vi "TableCnt.vi"(7 "cnt":T1, 8 "error in":errorcluster caption="에러 입력(에러 없음)", 10 "appended array":string[](array[string]), 11 "table_result":refnum<vi>) -> (0 "error out":errorcluster, 3 "Item Names":string[][](array[string]))   [LabVIEW 2019]
uses:
  cmd_tablecnt.ctl
  <vilib>/Utility/miscctls.llb/LVRowAndColumnTypeDef.ctl
  _ctrl/rw.ctl
  Durability/common/Global 1.vi
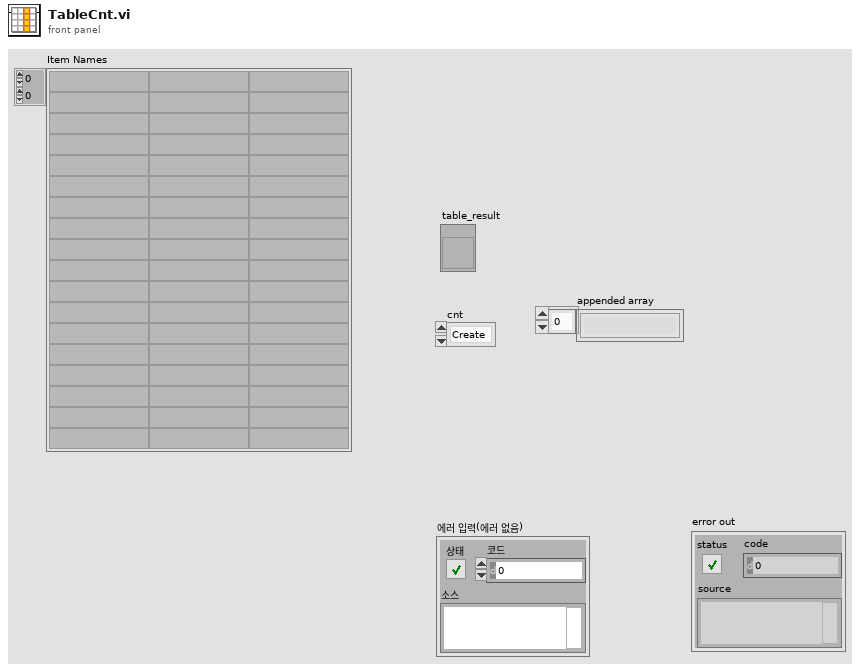
[diagram p1: front panel]
types:
  T1 = typedef "cmd_tablecnt.ctl" = enum16{"Create", "Inital", "Write", "Default"}
  T2 = typedef "LVRowAndColumnTypeDef.ctl" = cluster{"Row":i32, "Column":i32}
  T3 = typedef "rw.ctl" = enum16{"read", "write"}
  T4 = typedef "Test Mode.ctl" = enum32{"저항부하", "캐패시터부하", "B수명 - 1", "B수명 - 2", "B수명 - 3", "저전압모드 동작검사", "저전압모드 접촉저항", "고전압모드 동작검사"}
  T5 = typedef "Testing-info.ctl" = cluster{"전체채널수":u8, "현재채널번호":u8, "Irms":dbl, "입력전압":dbl, "입력전류":dbl, "출력전압":dbl, "출력전류":dbl, "온도":dbl, "제어단 단선":bool, "제어단 단락":bool, "제어단 특성변화":bool, "출력단 단선":bool, "출력단 단락":bool, "출력단 특성변화":bool, "출력단 전압":bool, "카운트 일치":bool, "Irms 판정":bool, "온도":bool, "테스트 회수":u32, "TestType":T6, "현재회수":u32, "Ch selection":cluster{"1ch":bool, "2ch":bool, "3ch":bool, "4ch":bool, "5ch":bool, "6ch":bool}, "반복":u32, "Path":path, "파일생성주기":u32, "start time":dbl, "stop time":dbl, "현재반복회수":u32, "NG":cluster{"입출력 카운트":bool, "출력전류RMS":bool}}
  T6 = typedef "sequence_single.ctl" = enum16{"Register", "RC", "B1", "B2", "B3", "Oper_LV", "Oper_HV", "ContR_LV"}
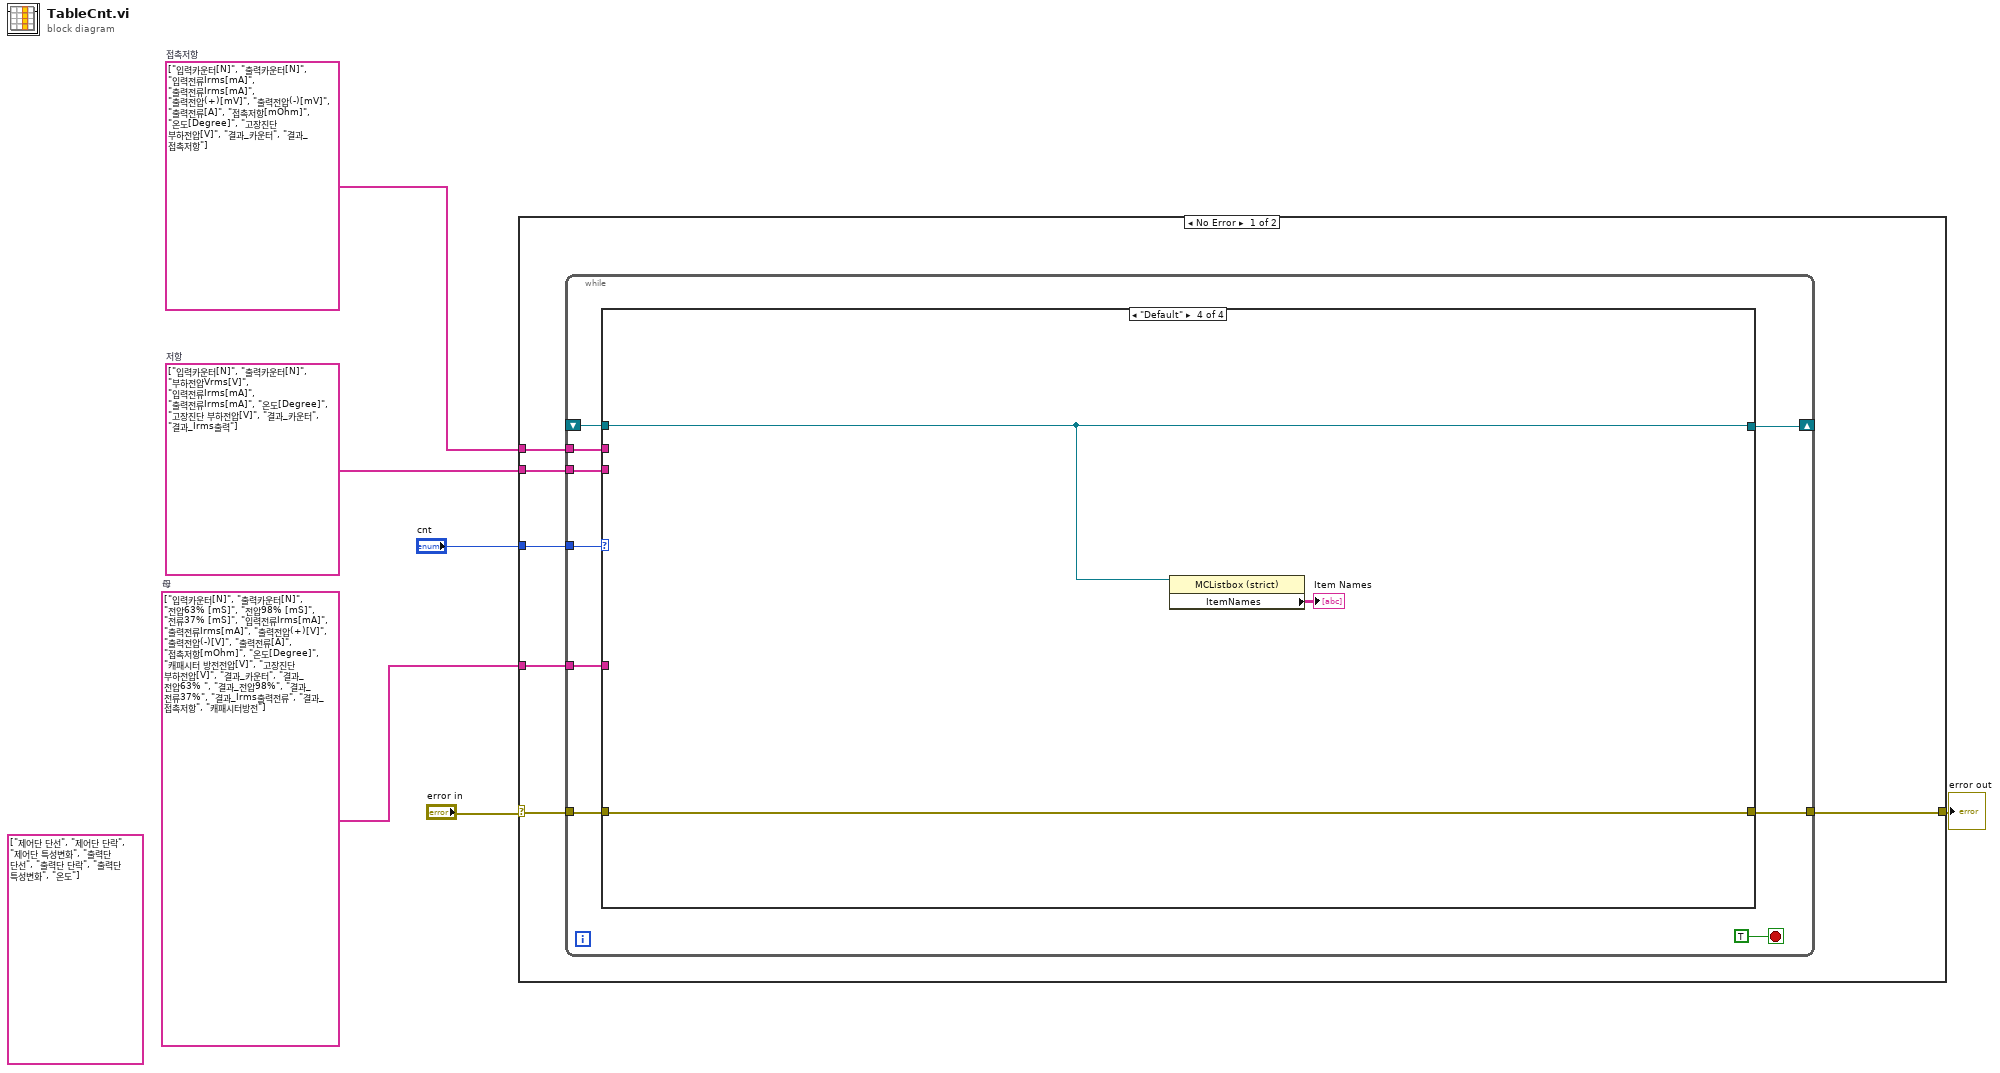
[diagram p0: block diagram]
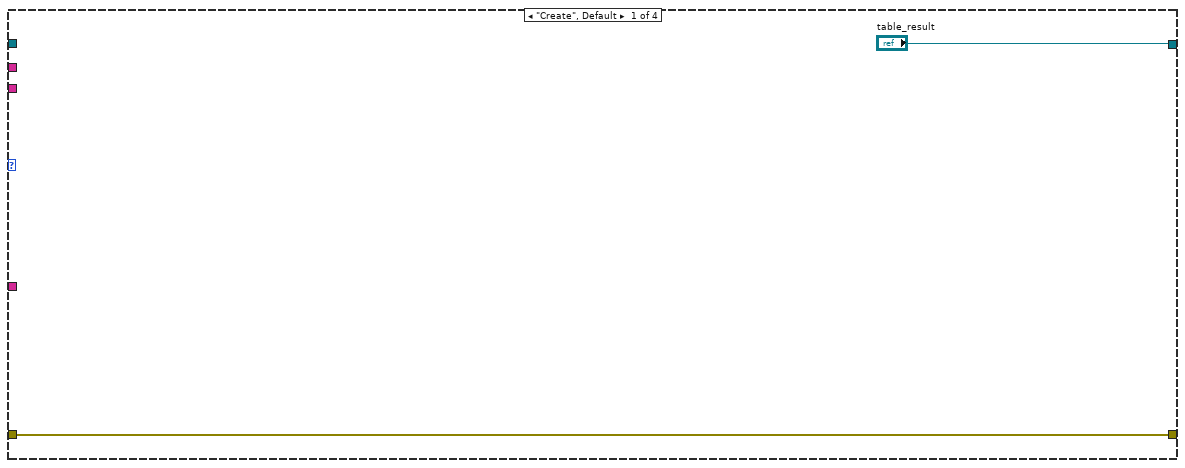
[diagram p2: hidden frame]
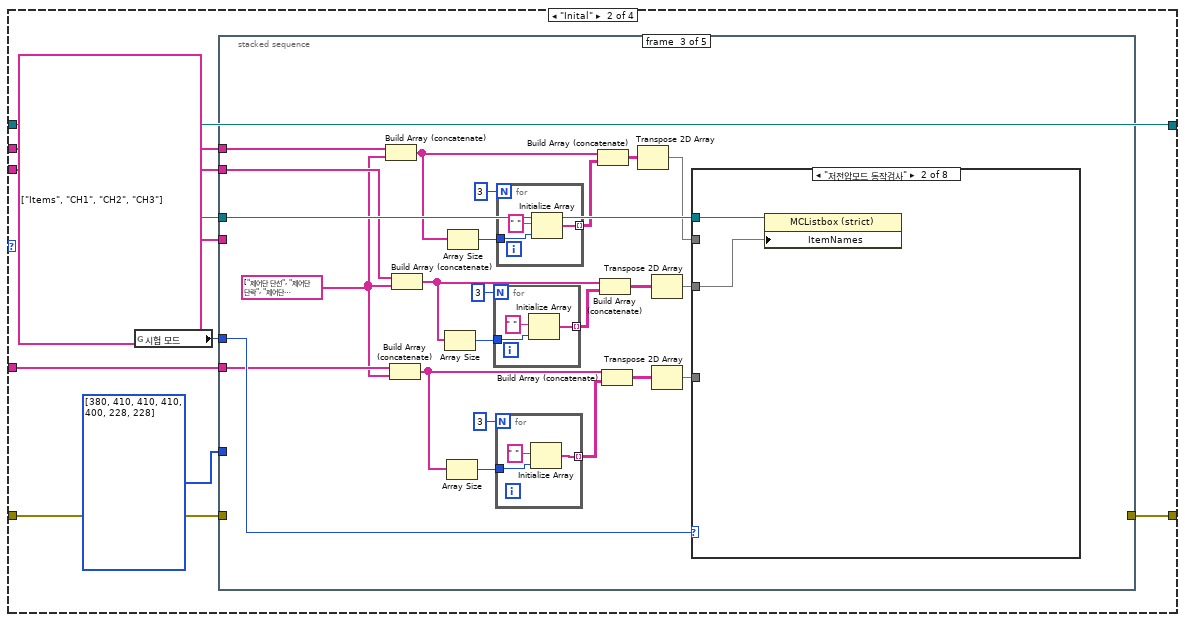
[diagram p3: hidden frame]
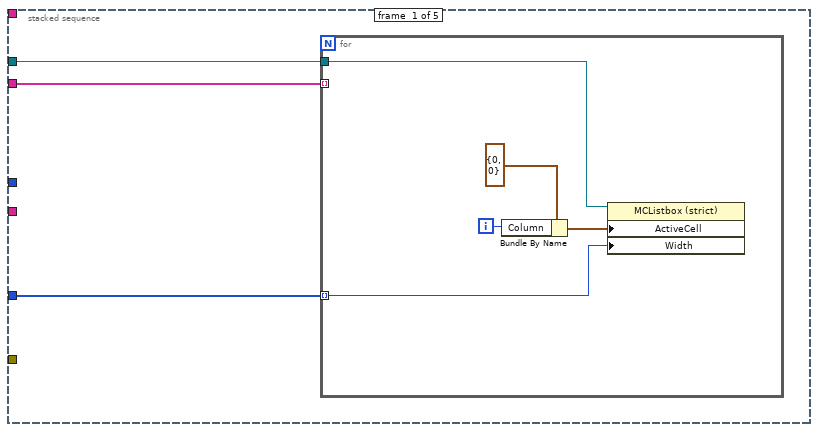
[diagram p4: hidden frame]
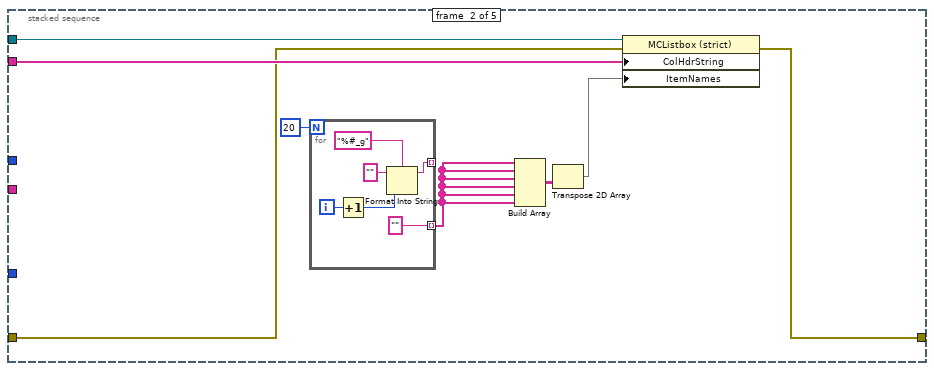
[diagram p5: hidden frame]
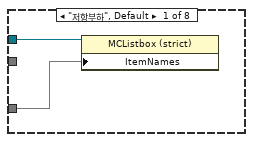
[diagram p6: hidden frame]
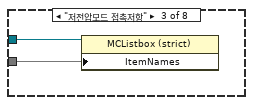
[diagram p7: hidden frame]
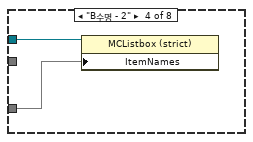
[diagram p8: hidden frame]
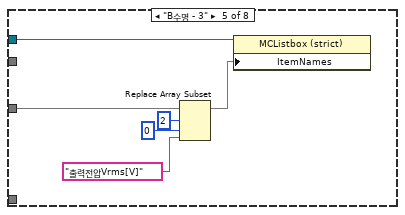
[diagram p9: hidden frame]
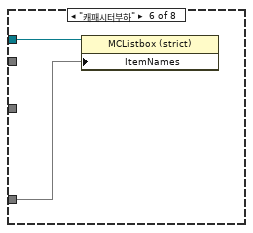
[diagram p10: hidden frame]
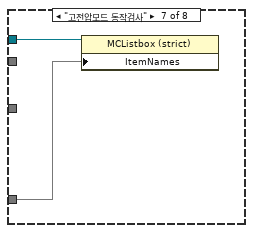
[diagram p11: hidden frame]
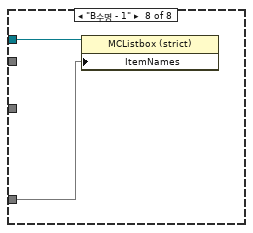
[diagram p12: hidden frame]
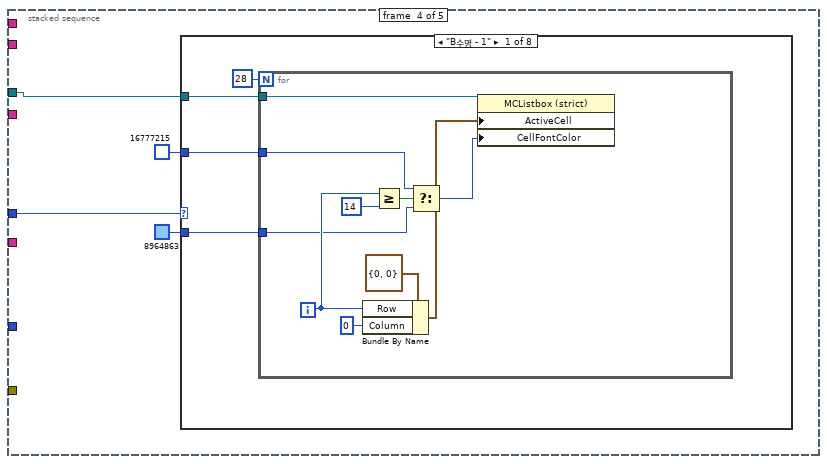
[diagram p13: hidden frame]
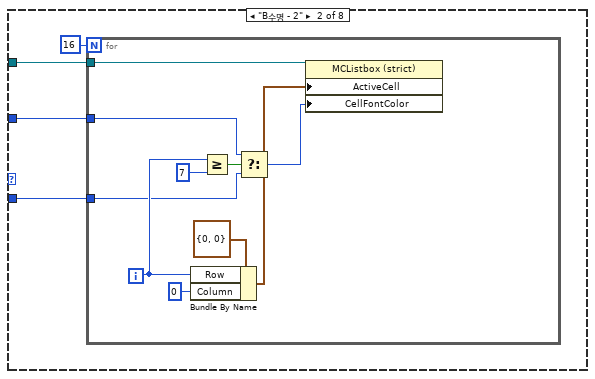
[diagram p14: hidden frame]
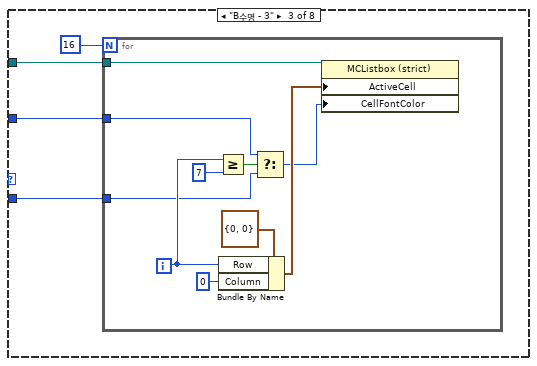
[diagram p15: hidden frame]
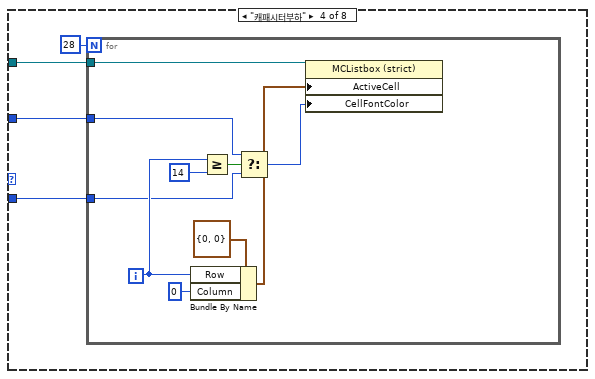
[diagram p16: hidden frame]
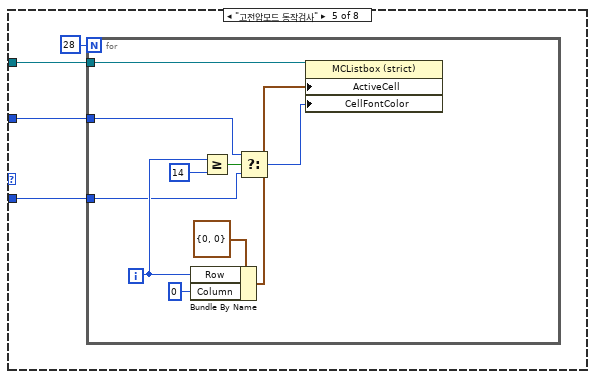
[diagram p17: hidden frame]
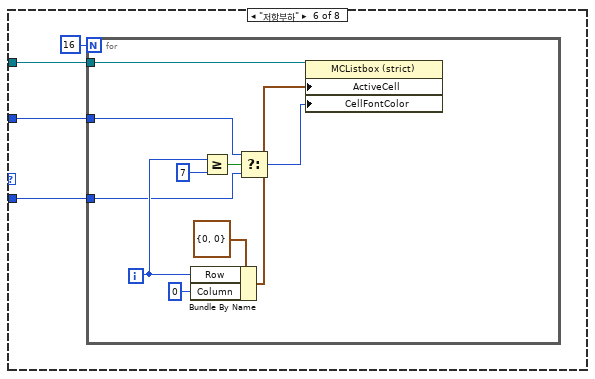
[diagram p18: hidden frame]
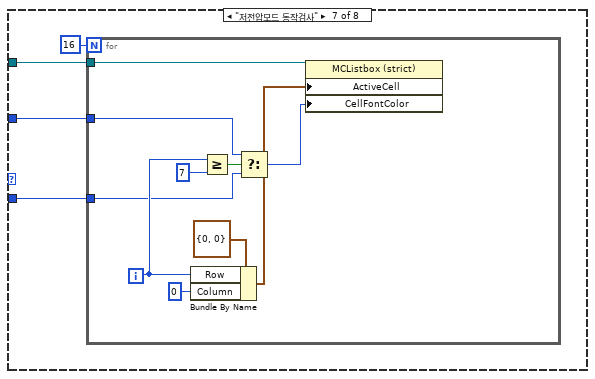
[diagram p19: hidden frame]
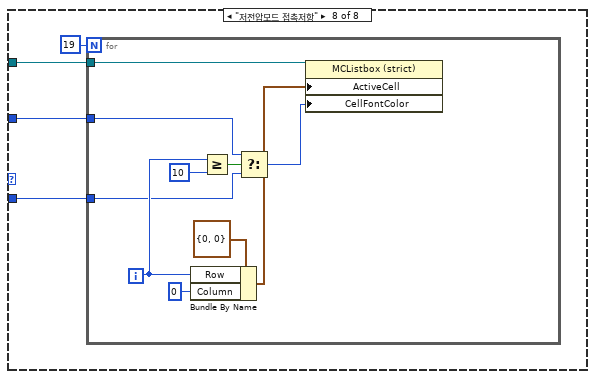
[diagram p20: hidden frame]
diagram:
  (unwired) string[] ["제어단 단선", "제어단 단락", "제어단 특성변화", "출력단 단선", "출력단 단락", "출력단 특성변화", "온도"] ("Column Header Strings[]")
  w1 = string[] ["입력카운터[N]", "출력카운터[N]", "입력전류Irms[mA]", "출력전류Irms[mA]", "출력전압(+)[mV]", "출력전압(-)[mV]", "출력전류[A]", "접촉저항[mOhm]", "온도[Degree]", "고장진단 부하전압[V]", "결과_카운터", "결과_접촉저항"]  # 접촉저항
  w2 = string[] ["입력카운터[N]", "출력카운터[N]", "전압63% [mS]", "전압98% [mS]", "전류37% [mS]", "입력전류Irms[mA]", "출력전류Irms[mA]", "출력전압(+)[V]", "출력전압(-)[V]", "출력전류[A]", "접촉저항[mOhm]", "온도[Degree]", "캐패시터 방전전압[V]", "고장진단 부하전압[V]", "결과_카운터", "결과_전압63% ", "결과_전압98%", "결과_전류37%", "결과_Irms출력전류", "결과_접촉저항", "캐패시터방전"]  # 母
  w3 = string[] ["입력카운터[N]", "출력카운터[N]", "부하전압Vrms[V]", "입력전류Irms[mA]", "출력전류Irms[mA]", "온도[Degree]", "고장진단 부하전압[V]", "결과_카운터", "결과_Irms출력"]  # 저항
  n1 = case shown="No Error" "error in" {
    selector: "error in" -> [w12 w443]
    tunnel: "cnt" -> [w11 _]
    tunnel: [w10 w443] -> w5
    tunnel: w3 -> [w9 _]
    tunnel: w2 -> [w8 _]
    tunnel: w1 -> [w7 _]
    frame No Error {
      n2 = while {
        tunnel: w12 -> [w17]
        tunnel: w11 -> [w20]
        shift-right: [w19] -> _
        shift-left: _ -> [w18]
        tunnel: [w16] -> w10
        tunnel: w9 -> [w15]
        tunnel: w8 -> [w14]
        tunnel: w7 -> [w13]
        stop <- TRUE stop-if-true
        n3 = case shown="\"Default\"" w20 {
          tunnel: ["table_result" w28 w227 w441] -> w19
          tunnel: w18 -> [_ w28 w227 w441]
          tunnel: w17 -> [w23 w31 _ w442]
          tunnel: [w23 w30 _ w442] -> w16
          tunnel: w15 -> [_ w26 _ _]
          tunnel: w14 -> [_ w25 _ _]
          tunnel: w13 -> [_ w24 _ _]
          frame "Create", Default {
          }
          frame "Inital" {
            n4 = global read "Global 1.vi" "시험 모드"() -> (w27:T4)
            n5 = stacked-sequence {
              tunnel: w28 -> [w34 w48 w78 w111 w225]
              tunnel: string[] ["Items", "CH1", "CH2", "CH3"] ("Column Header Strings[]") -> [w35 w47 _ _ _]
              tunnel: w31 -> [_ w46 _ _ _]
              tunnel: [_ w45 _ _ _] -> w30
              tunnel: u32[] [380, 410, 410, 410, 400, 228, 228] -> [w33 _ _ _ _]
              tunnel: w27 -> [_ _ w73 w110 _]
              tunnel: w26 -> [_ _ w64 _ _]
              tunnel: w25 -> [_ _ w63 _ _]
              tunnel: w24 -> [_ _ w61 _ _]
              frame #0 {
                n6 = for {
                  tunnel: w35 -> [_] mode=indexing
                  tunnel: w34 -> [w40]
                  tunnel: w33 -> [w37] mode=indexing
                  i -> [w36]
                  n7 = Bundle By Name(cluster=T2 {"Row"=0, "Column"=0} ("Active Cell:Active Cell"), "Column"=w36) -> (w38:T2)
                  n8 = property class="MCListbox (strict)"(reference=w40, "ActiveCell"=w38, "Width"=w37) -> ()  [unwired: 1 in, 2 out]
                }
              }
              frame #1 {
                n9 = for {
                  N: 20 -> [_]
                  tunnel: [w51] -> _ mode=indexing
                  tunnel: [""] -> w41 mode=indexing
                  i -> [w54]
                  n10 = Increment(x=w54) -> (x+1=w50:i32)
                  n11 = Format Into String(format string="%#_g" ("포맷 문자열"), initial string="" ("초기 문자열"), w50) -> (resulting string=w51:string)  [unwired: 1 in, 1 out]
                }
                n12 = Build Array(w41, w41, w41, w41, w41, w41) -> (w43:string[][])
                n13 = Transpose 2D Array(2D array=w43) -> (transposed array=w42:string[][])
                n14 = property class="MCListbox (strict)"(reference=w48, error in=w46, "ColHdrString"=w47, "ItemNames"=w42) -> (error out=w45:errorcluster)  [unwired: 1 out]
              }
              frame #2 {
                w62 = string[] ["제어단 단선", "제어단 단락", "제어단 특성변화", "출력단 단선", "출력단 단락", "출력단 특성변화", "온도"] ("Column Header Strings[]")
                n15 = Build Array (concatenate)(w61, w62) -> (w58:string[])
                n16 = Build Array (concatenate)(w63, w62) -> (w70:string[])
                n17 = Build Array (concatenate)(w64, w62) -> (w66:string[])
                n18 = Array Size(array=w66) -> (size(s)=w68:i32)
                n19 = Array Size(array=w70) -> (size(s)=w72:i32)
                n20 = Array Size(array=w58) -> (size(s)=w60:i32)
                n21 = for {
                  N: 3 -> [_]
                  tunnel: w68 -> [w83]
                  tunnel: [w82] -> w65 mode=indexing
                  n22 = Initialize Array(" ", w83) -> (w82:string[])
                }
                n23 = for {
                  N: 3 -> [_]
                  tunnel: w72 -> [w86]
                  tunnel: [w85] -> w69 mode=indexing
                  n24 = Initialize Array(" ", w86) -> (w85:string[])
                }
                n25 = for {
                  N: 3 -> [_]
                  tunnel: w60 -> [w80]
                  tunnel: [w79] -> w57 mode=indexing
                  n26 = Initialize Array(" ", w80) -> (w79:string[])
                }
                n27 = Build Array (concatenate)(w58, w57) -> (w56:string[][])
                n28 = Build Array (concatenate)(w66, w65) -> (w75:string[][])
                n29 = Build Array (concatenate)(w70, w69) -> (w74:string[][])
                n30 = Transpose 2D Array(2D array=w56) -> (transposed array=w55:string[][])
                n31 = Transpose 2D Array(2D array=w75) -> (transposed array=w77:string[][])
                n32 = Transpose 2D Array(2D array=w74) -> (transposed array=w76:string[][])
                n33 = case shown="\"저전압모드 동작검사\"" w73 {
                  tunnel: w78 -> [w89 w91 w93 w95 w101 w103 w105 w107]
                  tunnel: w77 -> [w88 w90 _ w94 w100 _ _ _]
                  tunnel: w76 -> [_ _ _ _ _ w102 w104 w106]
                  tunnel: w55 -> [_ _ w92 _ _ _ _ _]
                  frame "저항부하", Default {
                    n34 = property class="MCListbox (strict)"(reference=w89, "ItemNames"=w88) -> ()  [unwired: 1 in, 2 out]
                  }
                  frame "저전압모드 동작검사" {
                    n35 = property class="MCListbox (strict)"(reference=w91, "ItemNames"=w90) -> ()  [unwired: 1 in, 2 out]
                  }
                  frame "저전압모드 접촉저항" {
                    n36 = property class="MCListbox (strict)"(reference=w93, "ItemNames"=w92) -> ()  [unwired: 1 in, 2 out]
                  }
                  frame "B수명 - 2" {
                    n37 = property class="MCListbox (strict)"(reference=w95, "ItemNames"=w94) -> ()  [unwired: 1 in, 2 out]
                  }
                  frame "B수명 - 3" {
                    n38 = Replace Array Subset(array=w100, new element="출력전압Vrms[V]", index (row)=2, index (col)=0 ("disabled index (col)")) -> (w99:string[][])
                    n39 = property class="MCListbox (strict)"(reference=w101, "ItemNames"=w99) -> ()  [unwired: 1 in, 2 out]
                  }
                  frame "캐패시터부하" {
                    n40 = property class="MCListbox (strict)"(reference=w103, "ItemNames"=w102) -> ()  [unwired: 1 in, 2 out]
                  }
                  frame "고전압모드 동작검사" {
                    n41 = property class="MCListbox (strict)"(reference=w105, "ItemNames"=w104) -> ()  [unwired: 1 in, 2 out]
                  }
                  frame "B수명 - 1" {
                    n42 = property class="MCListbox (strict)"(reference=w107, "ItemNames"=w106) -> ()  [unwired: 1 in, 2 out]
                  }
                }
              }
              frame #3 {
                n43 = case shown="\"B수명 - 1\"" w110 {
                  tunnel: w111 -> [w115 w129 w143 w157 w171 w185 w199 w213]
                  tunnel: u32 16777215 -> [w113 w127 w141 w155 w169 w183 w197 w211]
                  tunnel: u32 8964863 -> [w112 w126 w140 w154 w168 w182 w196 w210]
                  frame "B수명 - 1" {
                    n44 = for {
                      N: 28 -> [_]
                      tunnel: w115 -> [w125]
                      tunnel: w113 -> [w117]
                      tunnel: w112 -> [w116]
                      i -> [w121]
                      n45 = Bundle By Name(cluster=T2 {"Row"=0, "Column"=0} ("Active Cell:Active Cell"), "Row"=w121, "Column"=0) -> (w123:T2)
                      n46 = Greater Or Equal?(x=w121, y=14 ("x")) -> (x >= y?=w119:bool)
                      n47 = Select(t=w117, s=w119, f=w116) -> (s? t:f=w118:u32)
                      n48 = property class="MCListbox (strict)"(reference=w125, "ActiveCell"=w123, "CellFontColor"=w118) -> ()  [unwired: 1 in, 2 out]
                    }
                  }
                  frame "B수명 - 2" {
                    n49 = for {
                      N: 16 -> [_]
                      tunnel: w129 -> [w139]
                      tunnel: w127 -> [w131]
                      tunnel: w126 -> [w130]
                      i -> [w135]
                      n50 = Bundle By Name(cluster=T2 {"Row"=0, "Column"=0} ("Active Cell:Active Cell"), "Row"=w135, "Column"=0) -> (w137:T2)
                      n51 = Greater Or Equal?(x=w135, y=7 ("x")) -> (x >= y?=w133:bool)
                      n52 = Select(t=w131, s=w133, f=w130) -> (s? t:f=w132:u32)
                      n53 = property class="MCListbox (strict)"(reference=w139, "ActiveCell"=w137, "CellFontColor"=w132) -> ()  [unwired: 1 in, 2 out]
                    }
                  }
                  frame "B수명 - 3" {
                    n54 = for {
                      N: 16 -> [_]
                      tunnel: w143 -> [w153]
                      tunnel: w141 -> [w145]
                      tunnel: w140 -> [w144]
                      i -> [w149]
                      n55 = Greater Or Equal?(x=w149, y=7 ("x")) -> (x >= y?=w147:bool)
                      n56 = Bundle By Name(cluster=T2 {"Row"=0, "Column"=0} ("Active Cell:Active Cell"), "Row"=w149, "Column"=0) -> (w151:T2)
                      n57 = Select(t=w145, s=w147, f=w144) -> (s? t:f=w146:u32)
                      n58 = property class="MCListbox (strict)"(reference=w153, "ActiveCell"=w151, "CellFontColor"=w146) -> ()  [unwired: 1 in, 2 out]
                    }
                  }
                  frame "캐패시터부하" {
                    n59 = for {
                      N: 28 -> [_]
                      tunnel: w157 -> [w167]
                      tunnel: w155 -> [w159]
                      tunnel: w154 -> [w158]
                      i -> [w163]
                      n60 = Bundle By Name(cluster=T2 {"Row"=0, "Column"=0} ("Active Cell:Active Cell"), "Row"=w163, "Column"=0) -> (w165:T2)
                      n61 = Greater Or Equal?(x=w163, y=14 ("x")) -> (x >= y?=w161:bool)
                      n62 = Select(t=w159, s=w161, f=w158) -> (s? t:f=w160:u32)
                      n63 = property class="MCListbox (strict)"(reference=w167, "ActiveCell"=w165, "CellFontColor"=w160) -> ()  [unwired: 1 in, 2 out]
                    }
                  }
                  frame "고전압모드 동작검사" {
                    n64 = for {
                      N: 28 -> [_]
                      tunnel: w171 -> [w181]
                      tunnel: w169 -> [w173]
                      tunnel: w168 -> [w172]
                      i -> [w177]
                      n65 = Bundle By Name(cluster=T2 {"Row"=0, "Column"=0} ("Active Cell:Active Cell"), "Row"=w177, "Column"=0) -> (w179:T2)
                      n66 = Greater Or Equal?(x=w177, y=14 ("x")) -> (x >= y?=w175:bool)
                      n67 = Select(t=w173, s=w175, f=w172) -> (s? t:f=w174:u32)
                      n68 = property class="MCListbox (strict)"(reference=w181, "ActiveCell"=w179, "CellFontColor"=w174) -> ()  [unwired: 1 in, 2 out]
                    }
                  }
                  frame "저항부하" {
                    n69 = for {
                      N: 16 -> [_]
                      tunnel: w185 -> [w195]
                      tunnel: w183 -> [w187]
                      tunnel: w182 -> [w186]
                      i -> [w191]
                      n70 = Bundle By Name(cluster=T2 {"Row"=0, "Column"=0} ("Active Cell:Active Cell"), "Row"=w191, "Column"=0) -> (w193:T2)
                      n71 = Greater Or Equal?(x=w191, y=7 ("x")) -> (x >= y?=w189:bool)
                      n72 = Select(t=w187, s=w189, f=w186) -> (s? t:f=w188:u32)
                      n73 = property class="MCListbox (strict)"(reference=w195, "ActiveCell"=w193, "CellFontColor"=w188) -> ()  [unwired: 1 in, 2 out]
                    }
                  }
                  frame "저전압모드 동작검사" {
                    n74 = for {
                      N: 16 -> [_]
                      tunnel: w199 -> [w209]
                      tunnel: w197 -> [w201]
                      tunnel: w196 -> [w200]
                      i -> [w205]
                      n75 = Bundle By Name(cluster=T2 {"Row"=0, "Column"=0} ("Active Cell:Active Cell"), "Row"=w205, "Column"=0) -> (w207:T2)
                      n76 = Greater Or Equal?(x=w205, y=7 ("x")) -> (x >= y?=w203:bool)
                      n77 = Select(t=w201, s=w203, f=w200) -> (s? t:f=w202:u32)
                      n78 = property class="MCListbox (strict)"(reference=w209, "ActiveCell"=w207, "CellFontColor"=w202) -> ()  [unwired: 1 in, 2 out]
                    }
                  }
                  frame "저전압모드 접촉저항" {
                    n79 = for {
                      N: 19 -> [_]
                      tunnel: w213 -> [w223]
                      tunnel: w211 -> [w215]
                      tunnel: w210 -> [w214]
                      i -> [w219]
                      n80 = Bundle By Name(cluster=T2 {"Row"=0, "Column"=0} ("Active Cell:Active Cell"), "Row"=w219, "Column"=0) -> (w221:T2)
                      n81 = Greater Or Equal?(x=w219, y=10 ("x")) -> (x >= y?=w217:bool)
                      n82 = Select(t=w215, s=w217, f=w214) -> (s? t:f=w216:u32)
                      n83 = property class="MCListbox (strict)"(reference=w223, "ActiveCell"=w221, "CellFontColor"=w216) -> ()  [unwired: 1 in, 2 out]
                    }
                  }
                }
              }
              frame #4 {
                n84 = property class="MCListbox (strict)"(reference=w225, "Value"=-1) -> ()  [unwired: 1 in, 2 out]
              }
            }
          }
          frame "Write" {
            n85 = property class="MCListbox (strict)"(reference=w227) -> ("ItemNames"=w230:string[][])  [unwired: 1 in, 2 out]
            n86 = global read "Global 1.vi" "시험 모드"() -> (w226:T4)
            n87 = call "fgv_curr-test-info.vi"("cmd"=rw."read") -> ("현재테스트 정보 2"=w229:T5)  [unwired: 10 in]
            n88 = case shown="\"저전압모드 접촉저항\"" w226 {
              tunnel: w230 -> [_ w240 w266 w292 w318 w344 w370 w396 w422]
              tunnel: w229 -> [_ w239 w265 w291 w317 w343 w369 w395 w421]
              tunnel: "appended array" -> [_ w236 w262 w288 w314 w340 w366 w392 w418]
              tunnel: w227 -> [_ w235 w261 w287 w313 w339 w365 w391 w417]
              frame Default {
              }
              frame "저항부하" {
                n89 = Unbundle By Name(w239) -> ("현재채널번호"=w232:u8)
                n90 = Increment(x=w232) -> (x+1=w237:u8)
                n91 = for {
                  tunnel: w236 -> [w243] mode=indexing
                  tunnel: [w241] -> w238 mode=indexing
                  n92 = Equal?(x=w243, y="NG") -> (x = y?=w241:bool)
                }
                n93 = Replace Array Subset(array=w240, new element=w236, index (col)=w237) -> (w233:string[][])  [unwired: 1 in]
                n94 = for {
                  tunnel: w235 -> [w257]
                  tunnel: w238 -> [w255] mode=indexing
                  tunnel: w237 -> [w251]
                  tunnel: w236 -> [_] mode=indexing
                  tunnel: [w244] -> w234
                  i -> [w250]
                  n95 = Select(t=u32 16711680, s=w255, f=u32 6618880) -> (s? t:f=w247:u32)
                  n96 = Greater Or Equal?(x=w250, y=7) -> (x >= y?=w248:bool)
                  n97 = Bundle By Name(cluster=T2 {"Row"=0, "Column"=0} ("Active Cell:Active Cell"), "Row"=w250, "Column"=w251) -> (w252:T2)
                  n98 = Select(t=w247, s=w248, f=u32 10537215) -> (s? t:f=w246:u32)
                  n99 = property class="MCListbox (strict)"(reference=w257, "ActiveCell"=w252, "CellFontColor"=w246) -> (reference out=w244:refnum<vi>)  [unwired: 1 in, 1 out]
                }
                n100 = property class="MCListbox (strict)"(reference=w234, "ItemNames"=w233) -> ()  [unwired: 1 in, 2 out]
              }
              frame "저전압모드 동작검사" {
                n101 = Unbundle By Name(w265) -> ("현재채널번호"=w258:u8)
                n102 = Increment(x=w258) -> (x+1=w263:u8)
                n103 = for {
                  tunnel: w262 -> [w269] mode=indexing
                  tunnel: [w267] -> w264 mode=indexing
                  n104 = Equal?(x=w269, y="NG") -> (x = y?=w267:bool)
                }
                n105 = Replace Array Subset(array=w266, new element=w262, index (col)=w263) -> (w259:string[][])  [unwired: 1 in]
                n106 = for {
                  tunnel: w261 -> [w283]
                  tunnel: w264 -> [w281] mode=indexing
                  tunnel: w263 -> [w277]
                  tunnel: w262 -> [_] mode=indexing
                  tunnel: [w270] -> w260
                  i -> [w276]
                  n107 = Select(t=u32 16711680, s=w281, f=u32 6618880) -> (s? t:f=w273:u32)
                  n108 = Greater Or Equal?(x=w276, y=7) -> (x >= y?=w274:bool)
                  n109 = Bundle By Name(cluster=T2 {"Row"=0, "Column"=0} ("Active Cell:Active Cell"), "Row"=w276, "Column"=w277) -> (w278:T2)
                  n110 = Select(t=w273, s=w274, f=u32 10537215) -> (s? t:f=w272:u32)
                  n111 = property class="MCListbox (strict)"(reference=w283, "ActiveCell"=w278, "CellFontColor"=w272) -> (reference out=w270:refnum<vi>)  [unwired: 1 in, 1 out]
                }
                n112 = property class="MCListbox (strict)"(reference=w260, "ItemNames"=w259) -> ()  [unwired: 1 in, 2 out]
              }
              frame "저전압모드 접촉저항" {
                n113 = Unbundle By Name(w291) -> ("현재채널번호"=w284:u8)
                n114 = Increment(x=w284) -> (x+1=w289:u8)
                n115 = for {
                  tunnel: w288 -> [w295] mode=indexing
                  tunnel: [w293] -> w290 mode=indexing
                  n116 = Equal?(x=w295, y="NG") -> (x = y?=w293:bool)
                }
                n117 = Replace Array Subset(array=w292, new element=w288, index (col)=w289) -> (w285:string[][])  [unwired: 1 in]
                n118 = for {
                  tunnel: w287 -> [w309]
                  tunnel: w290 -> [w307] mode=indexing
                  tunnel: w289 -> [w303]
                  tunnel: w288 -> [_] mode=indexing
                  tunnel: [w296] -> w286
                  i -> [w302]
                  n119 = Select(t=u32 16711680, s=w307, f=u32 6618880) -> (s? t:f=w299:u32)
                  n120 = Greater Or Equal?(x=w302, y=10) -> (x >= y?=w300:bool)
                  n121 = Bundle By Name(cluster=T2 {"Row"=0, "Column"=0} ("Active Cell:Active Cell"), "Row"=w302, "Column"=w303) -> (w304:T2)
                  n122 = Select(t=w299, s=w300, f=u32 10537215) -> (s? t:f=w298:u32)
                  n123 = property class="MCListbox (strict)"(reference=w309, "ActiveCell"=w304, "CellFontColor"=w298) -> (reference out=w296:refnum<vi>)  [unwired: 1 in, 1 out]
                }
                n124 = property class="MCListbox (strict)"(reference=w286, "ItemNames"=w285) -> ()  [unwired: 1 in, 2 out]
              }
              frame "고전압모드 동작검사" {
                n125 = Unbundle By Name(w317) -> ("현재채널번호"=w310:u8)
                n126 = Increment(x=w310) -> (x+1=w315:u8)
                n127 = for {
                  tunnel: w314 -> [w321] mode=indexing
                  tunnel: [w319] -> w316 mode=indexing
                  n128 = Equal?(x=w321, y="NG") -> (x = y?=w319:bool)
                }
                n129 = Replace Array Subset(array=w318, new element=w314, index (col)=w315) -> (w311:string[][])  [unwired: 1 in]
                n130 = for {
                  tunnel: w313 -> [w335]
                  tunnel: w316 -> [w333] mode=indexing
                  tunnel: w315 -> [w329]
                  tunnel: w314 -> [_] mode=indexing
                  tunnel: [w322] -> w312
                  i -> [w328]
                  n131 = Select(t=u32 16711680, s=w333, f=u32 6618880) -> (s? t:f=w325:u32)
                  n132 = Greater Or Equal?(x=w328, y=14) -> (x >= y?=w326:bool)
                  n133 = Bundle By Name(cluster=T2 {"Row"=0, "Column"=0} ("Active Cell:Active Cell"), "Row"=w328, "Column"=w329) -> (w330:T2)
                  n134 = Select(t=w325, s=w326, f=u32 10537215) -> (s? t:f=w324:u32)
                  n135 = property class="MCListbox (strict)"(reference=w335, "ActiveCell"=w330, "CellFontColor"=w324) -> (reference out=w322:refnum<vi>)  [unwired: 1 in, 1 out]
                }
                n136 = property class="MCListbox (strict)"(reference=w312, "ItemNames"=w311) -> ()  [unwired: 1 in, 2 out]
              }
              frame "캐패시터부하" {
                n137 = Unbundle By Name(w343) -> ("현재채널번호"=w336:u8)
                n138 = Increment(x=w336) -> (x+1=w341:u8)
                n139 = for {
                  tunnel: w340 -> [w347] mode=indexing
                  tunnel: [w345] -> w342 mode=indexing
                  n140 = Equal?(x=w347, y="NG") -> (x = y?=w345:bool)
                }
                n141 = Replace Array Subset(array=w344, new element=w340, index (col)=w341) -> (w337:string[][])  [unwired: 1 in]
                n142 = for {
                  tunnel: w339 -> [w361]
                  tunnel: w342 -> [w359] mode=indexing
                  tunnel: w341 -> [w355]
                  tunnel: w340 -> [_] mode=indexing
                  tunnel: [w348] -> w338
                  i -> [w354]
                  n143 = Select(t=u32 16711680, s=w359, f=u32 6618880) -> (s? t:f=w351:u32)
                  n144 = Greater Or Equal?(x=w354, y=14) -> (x >= y?=w352:bool)
                  n145 = Bundle By Name(cluster=T2 {"Row"=0, "Column"=0} ("Active Cell:Active Cell"), "Row"=w354, "Column"=w355) -> (w356:T2)
                  n146 = Select(t=w351, s=w352, f=u32 10537215) -> (s? t:f=w350:u32)
                  n147 = property class="MCListbox (strict)"(reference=w361, "ActiveCell"=w356, "CellFontColor"=w350) -> (reference out=w348:refnum<vi>)  [unwired: 1 in, 1 out]
                }
                n148 = property class="MCListbox (strict)"(reference=w338, "ItemNames"=w337) -> ()  [unwired: 1 in, 2 out]
              }
              frame "B수명 - 1" {
                n149 = Unbundle By Name(w369) -> ("현재채널번호"=w362:u8)
                n150 = Increment(x=w362) -> (x+1=w367:u8)
                n151 = for {
                  tunnel: w366 -> [w373] mode=indexing
                  tunnel: [w371] -> w368 mode=indexing
                  n152 = Equal?(x=w373, y="NG") -> (x = y?=w371:bool)
                }
                n153 = Replace Array Subset(array=w370, new element=w366, index (col)=w367) -> (w363:string[][])  [unwired: 1 in]
                n154 = for {
                  tunnel: w365 -> [w387]
                  tunnel: w368 -> [w385] mode=indexing
                  tunnel: w367 -> [w381]
                  tunnel: w366 -> [_] mode=indexing
                  tunnel: [w374] -> w364
                  i -> [w380]
                  n155 = Select(t=u32 16711680, s=w385, f=u32 6618880) -> (s? t:f=w377:u32)
                  n156 = Greater Or Equal?(x=w380, y=14) -> (x >= y?=w378:bool)
                  n157 = Bundle By Name(cluster=T2 {"Row"=0, "Column"=0} ("Active Cell:Active Cell"), "Row"=w380, "Column"=w381) -> (w382:T2)
                  n158 = Select(t=w377, s=w378, f=u32 10537215) -> (s? t:f=w376:u32)
                  n159 = property class="MCListbox (strict)"(reference=w387, "ActiveCell"=w382, "CellFontColor"=w376) -> (reference out=w374:refnum<vi>)  [unwired: 1 in, 1 out]
                }
                n160 = property class="MCListbox (strict)"(reference=w364, "ItemNames"=w363) -> ()  [unwired: 1 in, 2 out]
              }
              frame "B수명 - 2" {
                n161 = Unbundle By Name(w395) -> ("현재채널번호"=w388:u8)
                n162 = Increment(x=w388) -> (x+1=w393:u8)
                n163 = for {
                  tunnel: w392 -> [w399] mode=indexing
                  tunnel: [w397] -> w394 mode=indexing
                  n164 = Equal?(x=w399, y="NG") -> (x = y?=w397:bool)
                }
                n165 = Replace Array Subset(array=w396, new element=w392, index (col)=w393) -> (w389:string[][])  [unwired: 1 in]
                n166 = for {
                  tunnel: w391 -> [w413]
                  tunnel: w394 -> [w411] mode=indexing
                  tunnel: w393 -> [w407]
                  tunnel: w392 -> [_] mode=indexing
                  tunnel: [w400] -> w390
                  i -> [w406]
                  n167 = Select(t=u32 16711680, s=w411, f=u32 6618880) -> (s? t:f=w403:u32)
                  n168 = Greater Or Equal?(x=w406, y=7) -> (x >= y?=w404:bool)
                  n169 = Bundle By Name(cluster=T2 {"Row"=0, "Column"=0} ("Active Cell:Active Cell"), "Row"=w406, "Column"=w407) -> (w408:T2)
                  n170 = Select(t=w403, s=w404, f=u32 10537215) -> (s? t:f=w402:u32)
                  n171 = property class="MCListbox (strict)"(reference=w413, "ActiveCell"=w408, "CellFontColor"=w402) -> (reference out=w400:refnum<vi>)  [unwired: 1 in, 1 out]
                }
                n172 = property class="MCListbox (strict)"(reference=w390, "ItemNames"=w389) -> ()  [unwired: 1 in, 2 out]
              }
              frame "B수명 - 3" {
                n173 = Unbundle By Name(w421) -> ("현재채널번호"=w414:u8)
                n174 = Increment(x=w414) -> (x+1=w419:u8)
                n175 = for {
                  tunnel: w418 -> [w425] mode=indexing
                  tunnel: [w423] -> w420 mode=indexing
                  n176 = Equal?(x=w425, y="NG") -> (x = y?=w423:bool)
                }
                n177 = Replace Array Subset(array=w422, new element=w418, index (col)=w419) -> (w415:string[][])  [unwired: 1 in]
                n178 = for {
                  tunnel: w417 -> [w439]
                  tunnel: w420 -> [w437] mode=indexing
                  tunnel: w419 -> [w433]
                  tunnel: w418 -> [_] mode=indexing
                  tunnel: [w426] -> w416
                  i -> [w432]
                  n179 = Select(t=u32 16711680, s=w437, f=u32 6618880) -> (s? t:f=w429:u32)
                  n180 = Greater Or Equal?(x=w432, y=7) -> (x >= y?=w430:bool)
                  n181 = Bundle By Name(cluster=T2 {"Row"=0, "Column"=0} ("Active Cell:Active Cell"), "Row"=w432, "Column"=w433) -> (w434:T2)
                  n182 = Select(t=w429, s=w430, f=u32 10537215) -> (s? t:f=w428:u32)
                  n183 = property class="MCListbox (strict)"(reference=w439, "ActiveCell"=w434, "CellFontColor"=w428) -> (reference out=w426:refnum<vi>)  [unwired: 1 in, 1 out]
                }
                n184 = property class="MCListbox (strict)"(reference=w416, "ItemNames"=w415) -> ()  [unwired: 1 in, 2 out]
              }
            }
          }
          frame "Default" {
            n185 = property class="MCListbox (strict)"(reference=w441) -> ("ItemNames"=→"Item Names":string[][])  [unwired: 1 in, 2 out]
          }
        }
      }
    }
    frame Error {
    }
  }
  "error out" <- w5
